vi "GetTypes.vi"(0 "vi reference":refnum<vi>, 1 "controls or indicators":cluster{"Name":string, "Variant Data":variant}[](array[cluster])) -> (7 "types":T1(array[cluster]))   [LabVIEW 2015]
uses:
  <vilib>/Utility/Data Type/NI_Data Type.lvlib
panel:
  # "Get All Types"
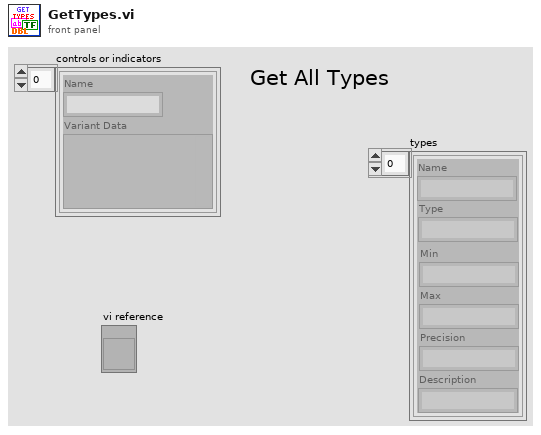
[diagram p1: front panel]
types:
  T1 = cluster{"Name":string, "Type":string, "Min":string, "Max":string, "Precision":string, "Description":string}[]
  T2 = cluster{"Name":string, "Type":string, "Min":string, "Max":string, "Precision":string, "Description":string}
  T3 = typedef "NI_Data Type.lvlib/Data Type.ctl" = enum8{"Invalid Type", "Void", "I8", "I16", "I32", "I64", "U8", "U16", "U32", "U64", "Single Float", "Double Float", "Extended Float", "Single Complex", "Double Complex", "Extended Complex", "Enum U8", "Enum U16", "Enum U32", "Enum U64", "Single Float With Unit", "Double Float With Unit", "Extended Float With Unit", "Single Complex with Unit", "Double Complex with Unit", "Extended Complex with Unit", "Boolean", "String", "Path", "Picture", "Tag", "Array", "Cluster", "Variant", "LV Variant", "Waveform", "Timestamp", "Digital Waveform", "Digital Data", "ExpressData", "Refnum", "External Data", "VI", "Poly VI", "LabVIEW Class Instance", "Fixed Point"}
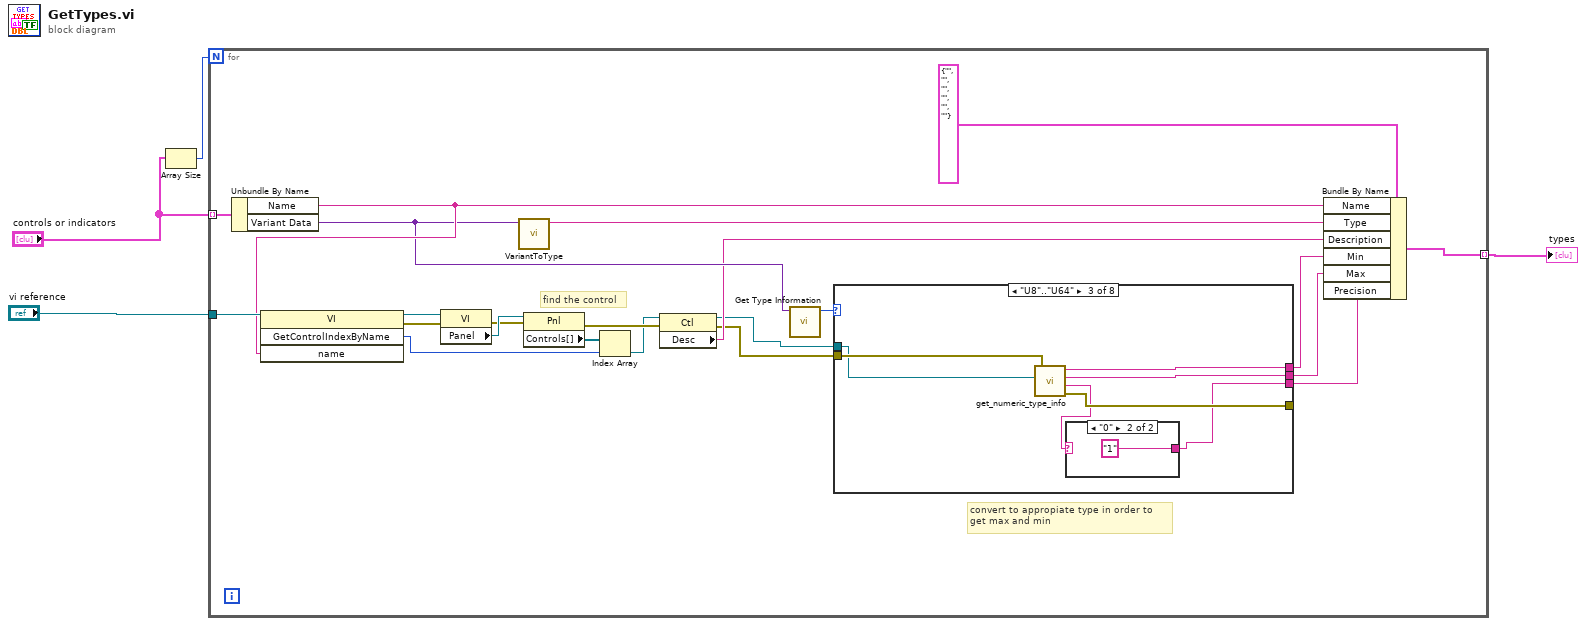
[diagram p0: block diagram]
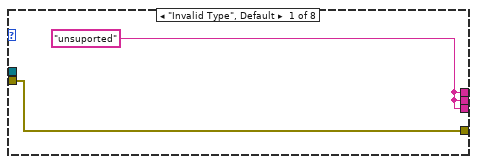
[diagram p2: hidden frame]
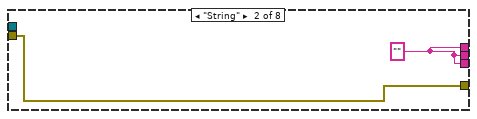
[diagram p3: hidden frame]
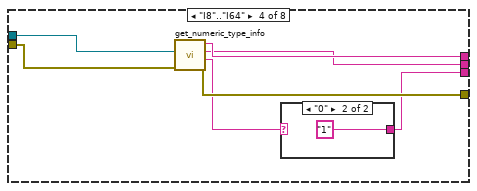
[diagram p5: hidden frame]
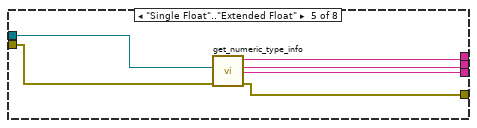
[diagram p7: hidden frame]
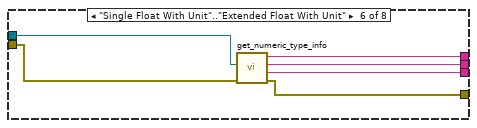
[diagram p8: hidden frame]
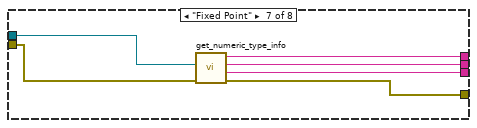
[diagram p9: hidden frame]
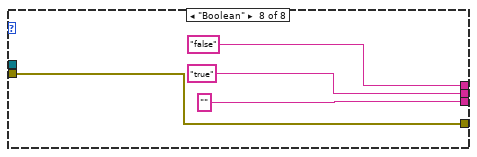
[diagram p10: hidden frame]
diagram:
  n1 = Array Size(array="controls or indicators") -> (size(s)=w4:i32)
  n2 = for {
    N: w4 -> [_]
    tunnel: "controls or indicators" -> [w26] mode=indexing
    tunnel: "vi reference" -> [w25]
    tunnel: [w16] -> w3 mode=indexing
    # "convert to appropiate type in order to \nget max and min"
    # "find the control"
    n3 = Unbundle By Name(w26) -> ("Name"=w24:string, "Variant Data"=w11:variant)
    n4 = invoke class="VI" method="GetControlIndexByName"(reference=w25, "name"=w24) -> (reference out=w23:refnum<vi>, error out=w19:errorcluster, "GetControlIndexByName"=w21:i32)  [unwired: 2 in, 1 out]
    n5 = property class="VI"(reference=w23, error in=w19) -> (error out=w18:errorcluster, "Panel"=w22:refnum<vi>)  [unwired: 1 out]
    n6 = call "VariantToType.vi"("Variant"=w11) -> ("type Name"=w15:string)  [unwired: 10 in]
    n7 = property class="Pnl"(reference=w22, error in=w18) -> (error out=w14:errorcluster, "Controls[]"=w20:refnum<vi>[])  [unwired: 1 out]
    n8 = Index Array(array=w20, index=w21) -> (element=w13:refnum<vi>)
    n9 = property class="Ctl"(reference=w13, error in=w14) -> (reference out=w8:refnum<vi>, error out=w9:errorcluster, "Desc"=w10:string)
    n10 = call <vilib>:"Get Type Information.vi"("Variant"=w11) -> ("Type"=w12:T3)  [unwired: 6 in, 4 out]
    n11 = case shown="\"U8\"..\"U64\"" w12 {
      tunnel: [w27 w30 w31 w40 w49 w58 w64 ""] -> w5
      tunnel: [w27 w30 w36 w45 w53 w59 w65 "true"] -> w6
      tunnel: [w27 w30 w37 w46 w54 w60 w66 "false"] -> w7
      tunnel: [w28 w29 w35 w44 w52 w57 w63 w67] -> _
      tunnel: w9 -> [w28 w29 w34 w42 w51 w55 w62 w67]
      tunnel: w8 -> [_ _ w33 w43 w50 w56 w61 _]
      frame "Invalid Type", Default {
        w27 = "unsuported"
      }
      frame "String" {
        w30 = "" ("Min")
      }
      frame "U8".."U64" {
        n12 = call "get_numeric_type_info.vi"("error in (no error)"=w34, "Refnum"=w33) -> ("error out"=w35:errorcluster, "Precision"=w32:string, "max"=w36:string, "Min"=w37:string)  [unwired: 6 in]
        n13 = case shown="\"0\"" w32 {
          selector: w32 -> [w38 _]
          tunnel: [w38 "1" ("Precision")] -> w31
          frame "False", Default {
          }
          frame "0" {
          }
        }
      }
      frame "I8".."I64" {
        n14 = call "get_numeric_type_info.vi"("error in (no error)"=w42, "Refnum"=w43) -> ("error out"=w44:errorcluster, "Precision"=w41:string, "max"=w45:string, "Min"=w46:string)  [unwired: 6 in]
        n15 = case shown="\"0\"" w41 {
          selector: w41 -> [w47 _]
          tunnel: [w47 "1" ("Precision")] -> w40
          frame "False", Default {
          }
          frame "0" {
          }
        }
      }
      frame "Single Float".."Extended Float" {
        n16 = call "get_numeric_type_info.vi"("error in (no error)"=w51, "Refnum"=w50) -> ("error out"=w52:errorcluster, "Precision"=w49:string, "max"=w53:string, "Min"=w54:string)  [unwired: 6 in]
      }
      frame "Single Float With Unit".."Extended Float With Unit" {
        n17 = call "get_numeric_type_info.vi"("error in (no error)"=w55, "Refnum"=w56) -> ("error out"=w57:errorcluster, "Precision"=w58:string, "max"=w59:string, "Min"=w60:string)  [unwired: 6 in]
      }
      frame "Fixed Point" {
        n18 = call "get_numeric_type_info.vi"("error in (no error)"=w62, "Refnum"=w61) -> ("error out"=w63:errorcluster, "Precision"=w64:string, "max"=w65:string, "Min"=w66:string)  [unwired: 6 in]
      }
      frame "Boolean" {
      }
    }
    n19 = Bundle By Name(cluster=T2 {"Name"="", "Type"="", "Min"="", "Max"="", "Precision"="", "Description"=""} ("element"), "Name"=w24, "Type"=w15, "Description"=w10, "Min"=w7, "Max"=w6, "Precision"=w5) -> (w16:T2)
  }
  "types" <- w3
